vi "TdmsReadLargeFile.vi"() -> ()   [LabVIEW 2011]
panel:
  in  "读取数目":i64=3
  out "数据":dbl[](array[numeric])
  in  "偏移量(0)":i64
  # "-1 表示全部读取, 显然对于大文件不能这么做,会内存不足"
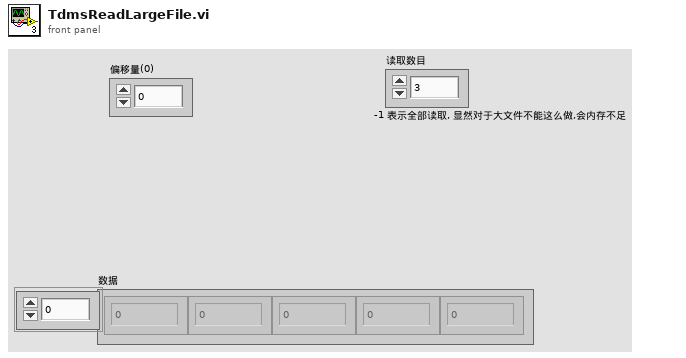
[diagram p1: front panel]
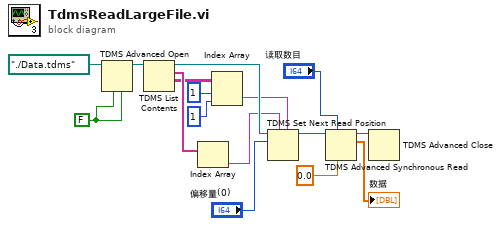
[diagram p0: block diagram]
diagram:
  w10 = FALSE ("禁用缓冲？(T)")
  n1 = TDMS Advanced Open(4:w10, 6:w10, 11:path "./Data.tdms" ("文件路径")) -> (3:w11:refnum<k34>)  [unwired: 2 in, 2 out]
  n2 = TDMS List Contents(7:w11) -> (1:w15:string[][], 2:w16:string[], 3:w9:refnum<k34>)  [unwired: 2 in, 1 out]
  n3 = Index Array(array=w16) -> (element=w8:string)  [unwired: 1 in]
  n4 = Index Array(array=w15, index (row)=1 ("索引 (行)"), index (col)=1 ("禁用的索引 (列)")) -> (element=w7:string)
  n5 = TDMS Set Next Read Position(5:w7, 7:w8, 10:"偏移量(0)", 11:w9) -> (3:w6:refnum<k34>)  [unwired: 2 in, 1 out]
  n6 = TDMS Advanced Synchronous Read(6:0.0, 7:"读取数目", 11:w6) -> (2:→"数据":dbl[], 3:w5:refnum<k34>)  [unwired: 1 in, 2 out]
  n7 = TDMS Advanced Close(11:w5) -> ()  [unwired: 3 in, 2 out]
